vi "pid_numerique_AhmedAmrani.vi"(4 "RAZ":bool, 6 "e_n":dbl, 7 "T":dbl, 9 "Td":dbl, 10 "Ti":dbl, 11 "Kp":dbl) -> (5 "u_n":dbl)   [LabVIEW 2012]
panel:
  out "Waveform Chart":cluster{"y_n":dbl, "e_n":dbl}(graph)={"y_n"=5.992595411754822, "e_n"=1.0}
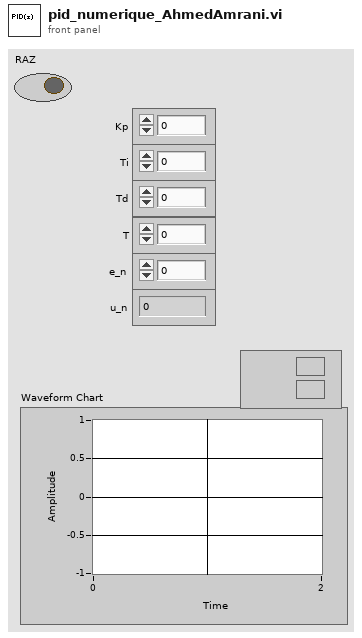
[diagram p1: front panel]
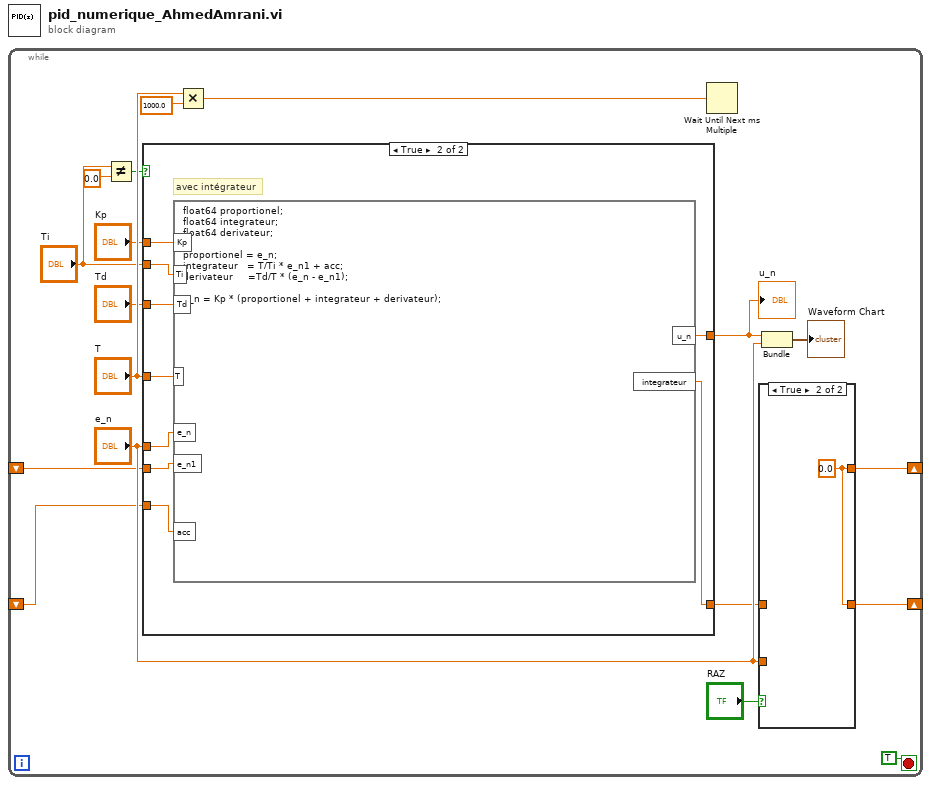
[diagram p0: block diagram]
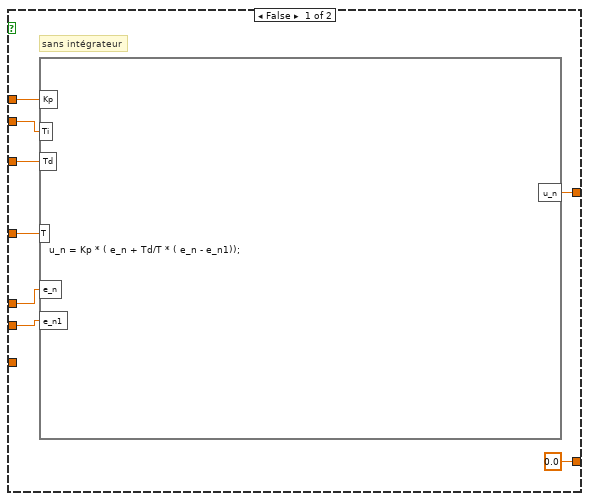
[diagram p3: hidden frame]
diagram:
  n1 = while {
    shift-right: [w5] -> _
    shift-left: _ -> [w4]
    shift-right: [w1] -> _
    shift-left: _ -> [w3]
    stop <- TRUE stop-if-true
    n2 = Not Equal?(x="Ti", y=0.0) -> (x != y?=w6:bool)
    n3 = case shown="True" w6 {
      tunnel: "Kp" -> [w28 w38]
      tunnel: "Ti" -> [w27 w37]
      tunnel: "Td" -> [w26 w36]
      tunnel: "T" -> [w25 w35]
      tunnel: "e_n" -> [w24 w34]
      tunnel: [w29 w33] -> w9
      tunnel: w4 -> [w23 w32]
      tunnel: [0.0 w31] -> w2
      tunnel: w3 -> [_ w30]
      frame False {
        # "sans intégrateur"
        n4 = formula code="u_n = Kp * ( e_n + Td/T * ( e_n - e_n1));"("Kp"=w28, "Ti"=w27, "Td"=w26, "T"=w25, "e_n"=w24, "e_n1"=w23) -> ("u_n"=w29:dbl)
      }
      frame True {
        # "avec intégrateur"
        n5 = formula code="float64 proportionel;\nfloat64 integrateur;\nfloat64 derivateur;\n\nproportionel = e_n;\nintegrateur   = T/Ti * e_n1 + acc;\nderivateur     =Td/T * (e_n - e_n1);\n\nu_n = Kp * (proportionel + integrateur + derivateur);"("Kp"=w38, "Ti"=w37, "Td"=w36, "T"=w35, "e_n"=w34, "e_n1"=w32, "acc"=w30) -> ("u_n"=w33:dbl, "integrateur"=w31:dbl)
      }
    }
    "u_n" <- w9
    n6 = Multiply(x="T", y=1000.0) -> (x*y=w15:dbl)
    n7 = Wait Until Next ms Multiple(millisecond multiple=w15) -> ()  [unwired: 1 out]
    n8 = case shown="True" "RAZ" {
      tunnel: [w20 w21] -> w5
      tunnel: "e_n" -> [w20 _]
      tunnel: w2 -> [w19 _]
      tunnel: [w19 w21] -> w1
      frame False {
      }
      frame True {
        w21 = 0.0 ("y_n")
      }
    }
    n9 = Bundle("u_n"=w9, "e_n"="e_n") -> (→"Waveform Chart":cluster{"u_n":dbl, "e_n":dbl})  [unwired: 1 in]
  }
